vi "Systemlink_ErrorCheck.vi"(11 "HTTP Code":i32) -> ()   [LabVIEW 2016, in "Systemlink Tag.xctl"]
uses:
  Systemlink Tag.xctl
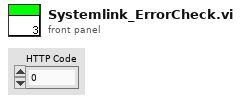
[diagram p1: front panel]
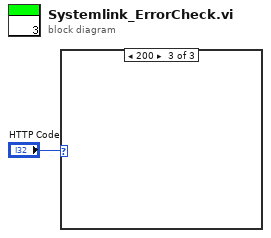
[diagram p0: block diagram]
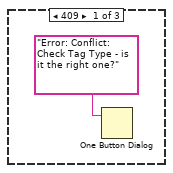
[diagram p2: hidden frame]
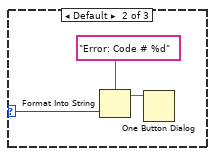
[diagram p3: hidden frame]
diagram:
  n1 = case shown="200" "HTTP Code" {
    selector: "HTTP Code" -> [_ w5 _]
    frame 409 {
      n2 = One Button Dialog(message="Error: Conflict: Check Tag Type - is it the right one?") -> ()  [unwired: 1 in, 1 out]
    }
    frame Default {
      n3 = Format Into String(format string="Error: Code # %d" ("message"), w5) -> (resulting string=w3:string)  [unwired: 2 in, 1 out]
      n4 = One Button Dialog(message=w3) -> ()  [unwired: 1 in, 1 out]
    }
    frame 200 {
    }
  }
